vi "8byte to 4 2byte.vi"(10 "payload":u8[](array[numeric])) -> (0 "7,6":i16, 1 "5,4":i16, 2 "3,2":i16, 3 "1,0":i16)   [LabVIEW 2015]
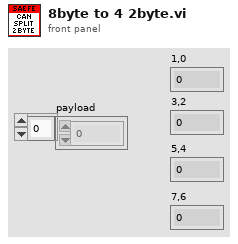
[diagram p1: front panel]
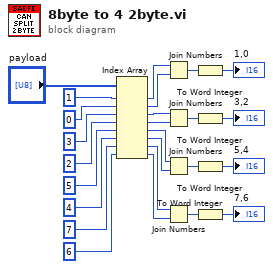
[diagram p0: block diagram]
diagram:
  n1 = Index Array(array="payload", index #1=1 ("index"), index #2=0 ("index"), index #3=3 ("index"), index #4=2 ("index"), index #5=5 ("index"), index #6=4 ("index"), index #7=7 ("index"), index #8=6 ("index")) -> (element #1=w18:u8, element #2=w19:u8, element #3=w20:u8, element #4=w21:u8, element #5=w22:u8, element #6=w23:u8, element #7=w24:u8, element #8=w25:u8)
  n2 = Join Numbers(hi=w18, lo=w19) -> ((hi.lo)=w2:u16)
  n3 = Join Numbers(hi=w20, lo=w21) -> ((hi.lo)=w4:u16)
  n4 = Join Numbers(hi=w22, lo=w23) -> ((hi.lo)=w6:u16)
  n5 = Join Numbers(hi=w24, lo=w25) -> ((hi.lo)=w8:u16)
  n6 = To Word Integer(number=w2) -> (16bit integer=→"1,0":i16)
  n7 = To Word Integer(number=w4) -> (16bit integer=→"3,2":i16)
  n8 = To Word Integer(number=w6) -> (16bit integer=→"5,4":i16)
  n9 = To Word Integer(number=w8) -> (16bit integer=→"7,6":i16)
